vi "Read SensorInfo.vi"(8 "error in (no error)":errorcluster, 11 "SensorCharm in":refnum<class "SensorCharm.lvclass">) -> (0 "error out":errorcluster, 2 "Sensor Definition.lvlib:SensorInfo.lvclass":refnum<class "SensorInfo.lvclass">, 3 "SensorCharm out":refnum<class "SensorCharm.lvclass">)   [LabVIEW 2012, in "Sensor Definition.lvlib" / "SensorCharm.lvclass"]
uses:
  SensorCharm.lvclass
  SensorInfo.lvclass
  SensorCharm.lvclass/SensorCharm.ctl
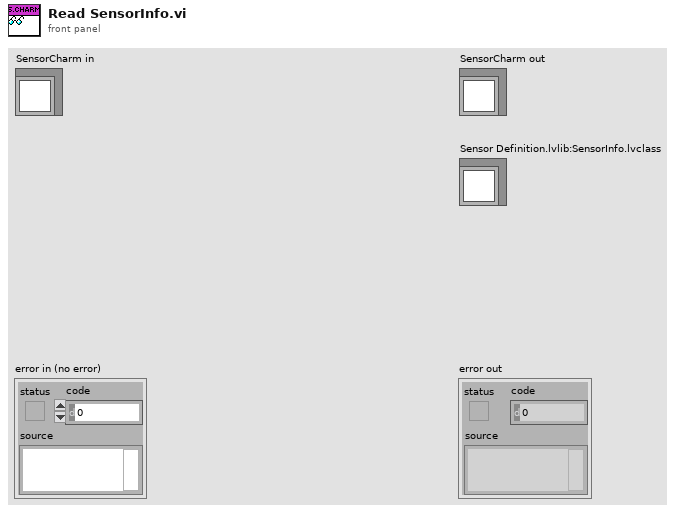
[diagram p1: front panel]
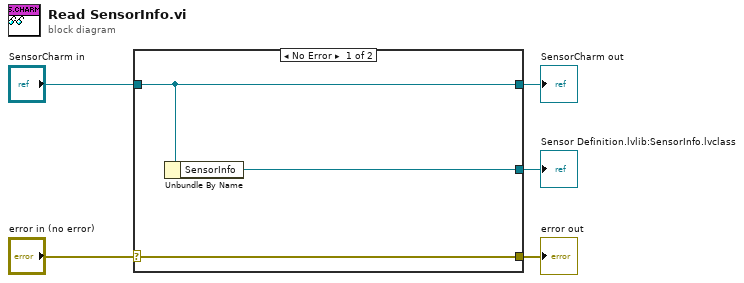
[diagram p0: block diagram]
diagram:
  n1 = case shown="No Error" "error in (no error)" {
    selector: "error in (no error)" -> [w8 w9]
    tunnel: [w8 w9] -> w4
    tunnel: [w7 w10] -> w2
    tunnel: "SensorCharm in" -> [w7 w10]
    tunnel: [w6 _] -> w1
    frame No Error {
      n2 = Unbundle By Name(w7) -> ("SensorInfo"=w6:refnum<class "SensorInfo.lvclass">)
    }
    frame Error {
    }
  }
  "error out" <- w4
  "SensorCharm out" <- w2
  "Sensor Definition.lvlib:SensorInfo.lvclass" <- w1
